vi "Destroy user events.vi"(8 "error in (no error)":errorcluster, 11 "User events":T1) -> (0 "error out":errorcluster)   [LabVIEW 2020, in "NI DAQ.lvlib"]
uses:
  NI DAQ.lvlib
  Task list.ctl
  Continuous aquisition params.ctl
  Controls/Acuisition type --typedef.ctl
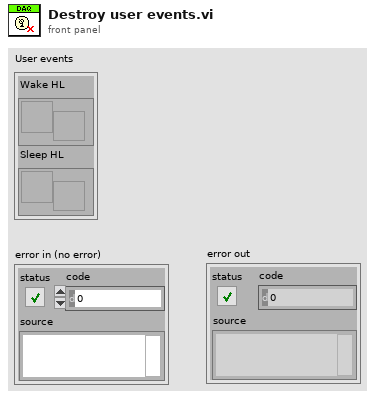
[diagram p1: front panel]
types:
  T1 = cluster{"Wake HL":refnum<user-event>, "Sleep HL":refnum<user-event>}
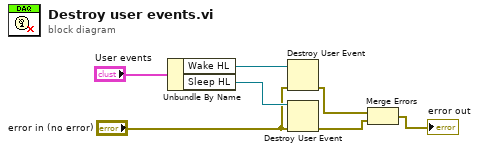
[diagram p0: block diagram]
diagram:
  n1 = Unbundle By Name("User events") -> ("Wake HL"=w6:refnum<user-event>, "Sleep HL"=w7:refnum<user-event>)
  n2 = Destroy User Event(user event=w6, error in="error in (no error)") -> (error out=w3:errorcluster)
  n3 = Destroy User Event(user event=w7, error in="error in (no error)") -> (error out=w2:errorcluster)
  n4 = Merge Errors(w3, w2) -> (→"error out":errorcluster)
